vi "CalcPerimiter.vi"(7 "Garden":u8[][](array[numeric]), 11 "Cluster":T1) -> (3 "Numeric":u64)   [LabVIEW 2023, in "2024_12.lvclass"]
uses:
  2024_12.lvclass
panel:
  out "Array":bool[][](array[boolean])
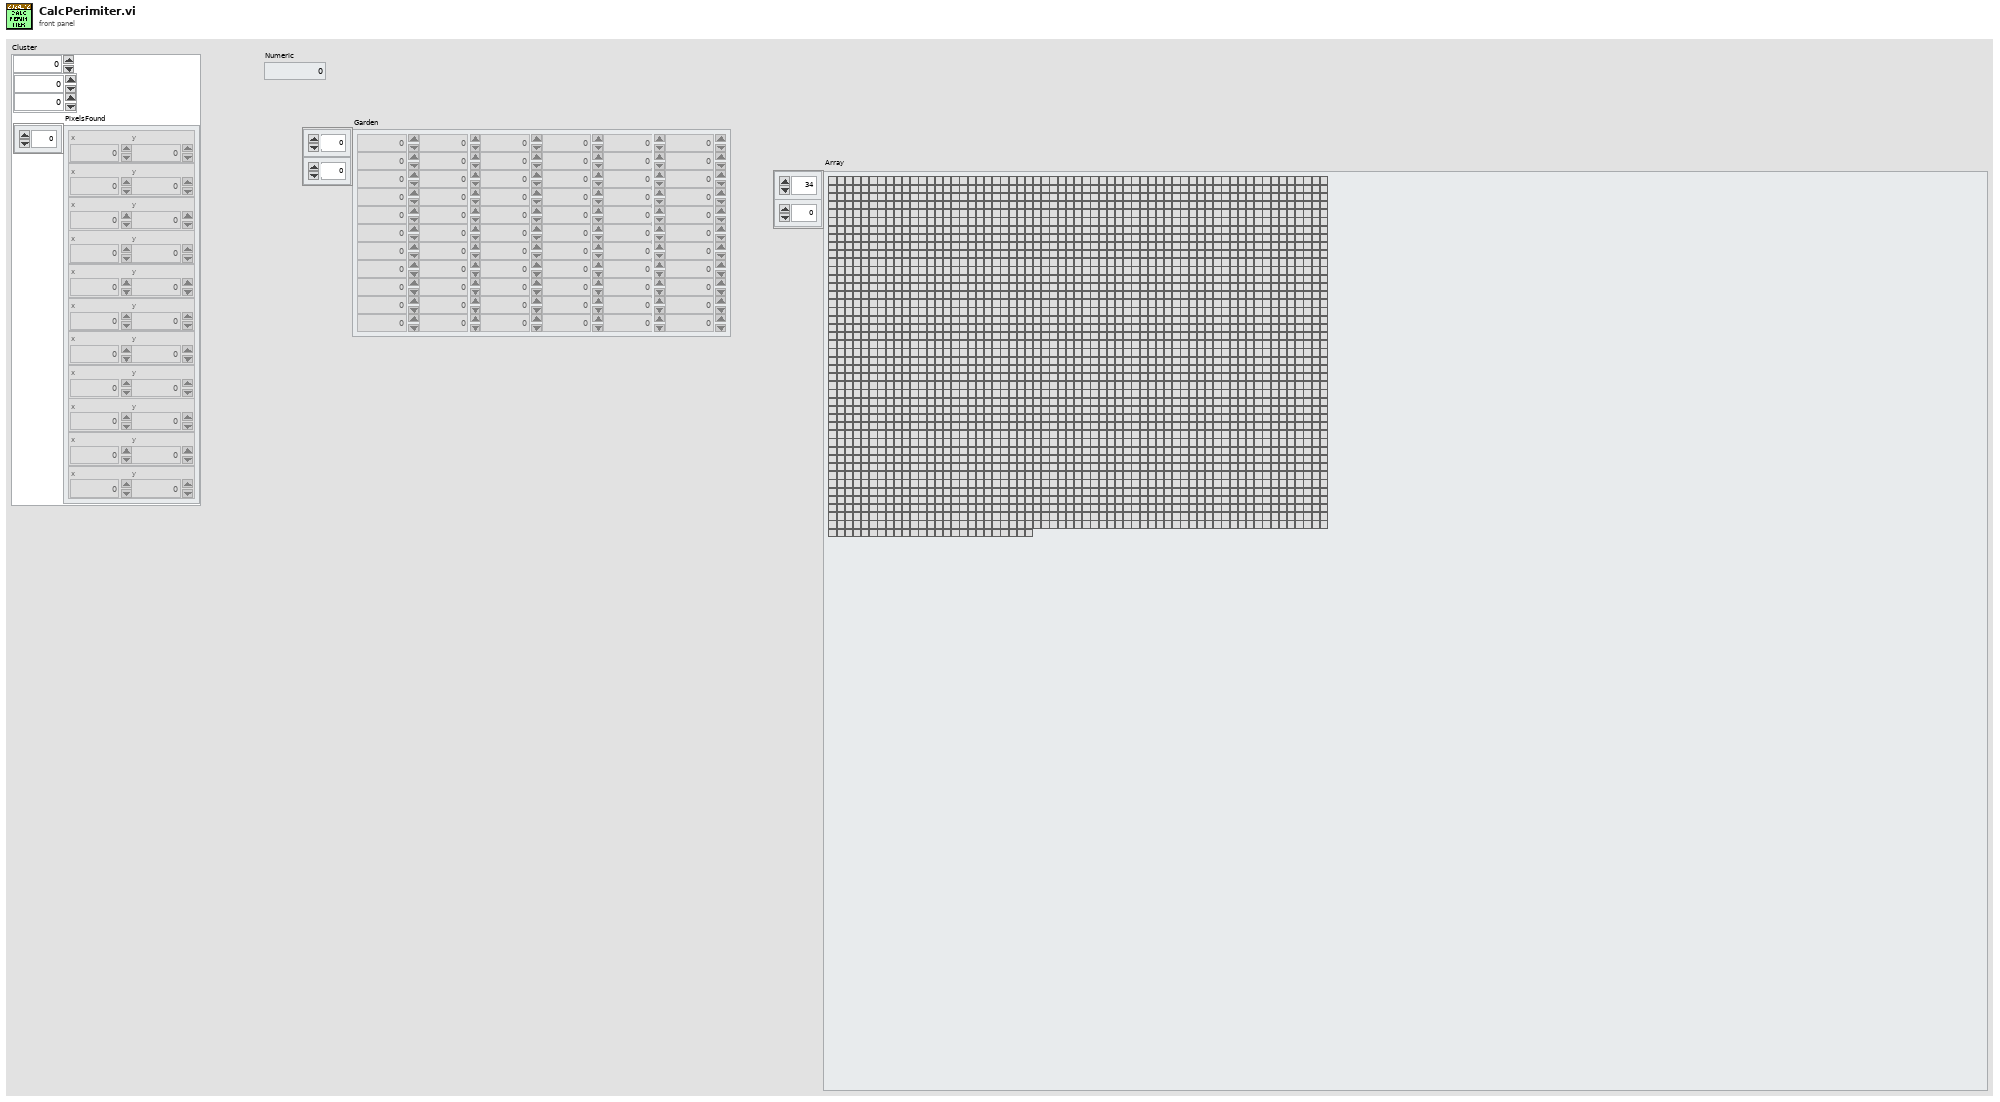
[diagram p1: front panel]
types:
  T1 = cluster{"Numeric":u8, "Cluster":cluster{"Numeric":i32, "Numeric":i32}, "PixelsFound":cluster{"x":i32, "y":i32}[]}
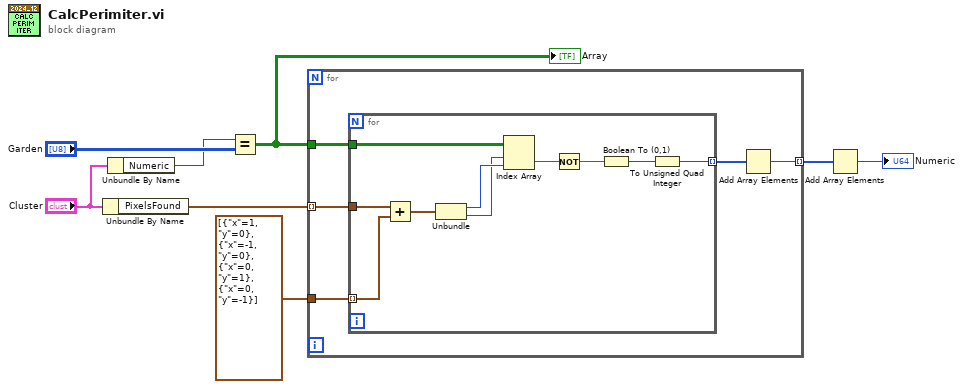
[diagram p0: block diagram]
diagram:
  n1 = Unbundle By Name("Cluster") -> ("PixelsFound"=w8:cluster{"x":i32, "y":i32}[])
  n2 = Unbundle By Name("Cluster") -> ("Numeric"=w5:u8)
  n3 = Equal?(x=w5, y="Garden") -> (x = y?=w1:bool[][])
  "Array" <- w1
  n4 = for {
    tunnel: w8 -> [w12] mode=indexing
    tunnel: w1 -> [w13]
    tunnel: cluster{"x":i32, "y":i32}[] [{"x"=1, "y"=0}, {"x"=-1, "y"=0}, {"x"=0, "y"=1}, {"x"=0, "y"=-1}] ("PixelsFound") -> [w11]
    tunnel: [w9] -> w3 mode=indexing
    n5 = for {
      tunnel: w13 -> [w23]
      tunnel: w12 -> [w22]
      tunnel: w11 -> [w21] mode=indexing
      tunnel: [w14] -> w10 mode=indexing
      n6 = Add(x=w22, y=w21) -> (x+y=w20:cluster{"x":i32, "y":i32})
      n7 = Unbundle(w20) -> ("x"=w19:i32, "y"=w18:i32)
      n8 = Index Array(array=w23, index (row)=w18, index (col)=w19) -> (element=w17:bool)
      n9 = Not(x=w17) -> (.not. x?=w16:bool)
      n10 = Boolean To (0,1)(Boolean=w16) -> (0, 1=w15:i16)
      n11 = To Unsigned Quad Integer(1:w15) -> (0:w14:u64)
    }
    n12 = Add Array Elements(numeric array=w10) -> (sum=w9:u64)
  }
  n13 = Add Array Elements(numeric array=w3) -> (sum=→"Numeric":u64)
